vi "Get Result.vi"(4 "Controller name":string, 6 "Last request":bool, 8 "error in (no error)":errorcluster, 11 "Instrument Recorder in":refnum<class "Stepper.lvclass">) -> (0 "error out":errorcluster, 2 "Result":refnum<class "Acquired Result.lvclass">, 3 "Instrument Recorder out":refnum<class "Stepper.lvclass">)   [LabVIEW 2021]
uses:
  Stepper.lvclass
  NHMFL_Core/Libraries/Instruments/Results/Acquired Result/Acquired Result.lvclass
  NHMFL_Core/Libraries/Instruments/Results/Combined Result/Combined Result.lvclass
  C:/Git/NHMFL_Core/Libraries/Instruments/Results/Acquired Result/Acquired Result.lvclass
  NHMFL_Core/Libraries/Instruments/Results/Acquired Result/Acquired Result.lvclass/Acquired Result.ctl
  NHMFL_Core/Libraries/Instruments/Results/Acquired Result/Write Group.vi
  Combined Measurement/Combined Measurement.lvclass
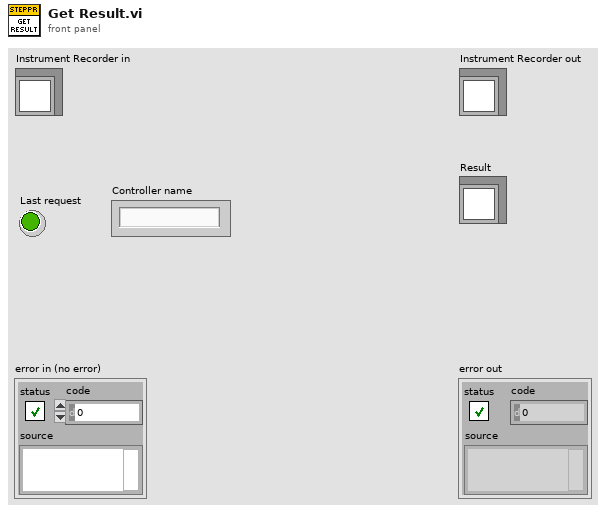
[diagram p1: front panel]
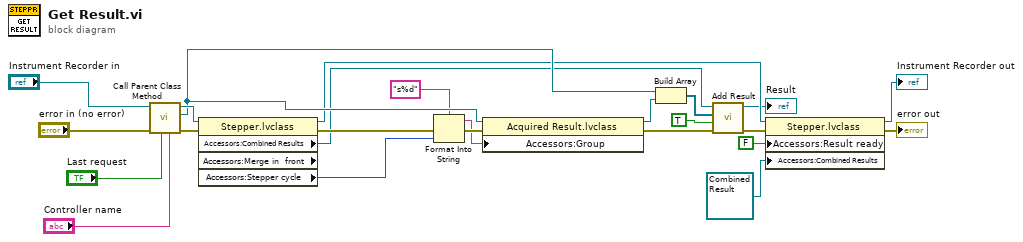
[diagram p0: block diagram]
diagram:
  n1 = call-parent "Call Parent Class Method"("Controller name"="Controller name", "Last request"="Last request", "error in (no error)"="error in (no error)", "Instrument Recorder in"="Instrument Recorder in") -> ("error out"=w24:errorcluster, "Result"=w18:refnum<class "Acquired Result.lvclass">, "Instrument Recorder out"=w19:refnum<class "Stepper.lvclass">)  [unwired: 5 in]
  n2 = property class="Stepper.lvclass" props=["Accessors:Combined Results", "Accessors:Merge in  front", "Accessors:Stepper cycle"](reference=w19, error in=w24) -> (reference out=w15:refnum<class "Stepper.lvclass">, error out=w17:errorcluster, "Accessors:Combined Results"=w8:refnum<class "Combined Result.lvclass">, "Accessors:Stepper cycle"=w11:i32)  [unwired: 1 out]
  n3 = Format Into String(format string="s%d", error in=w17, w11) -> (resulting string=w9:string, error out=w12:errorcluster)  [unwired: 1 in]
  n4 = property class="Acquired Result.lvclass"(reference=w18, error in=w12, "Accessors:Group"=w9) -> (reference out=w7:refnum<class "Acquired Result.lvclass">, error out=w4:errorcluster)
  n5 = Build Array(w18, w7) -> (w6:refnum<class "Acquired Result.lvclass">[])
  n6 = call-dynamic "Add Result.vi"("error in (no error)"=w4, "Add in front"=TRUE, "Results to add"=w6, "Combined Result in"=w8) -> ("error out"=w2:errorcluster, "Combined Result out"=→"Result":refnum<class "Combined Result.lvclass">)  [unwired: 6 in]
  n7 = property class="Stepper.lvclass"(reference=w15, error in=w2, "Accessors:Result ready"=FALSE ("Result ready"), "Accessors:Combined Results"=refnum<class "Combined Result.lvclass"> refnum ("Combined Results")) -> (reference out=→"Instrument Recorder out":refnum<class "Stepper.lvclass">, error out=→"error out":errorcluster)
